vi "Write to Spreadsheet File.vi"(7 "1D data":dbl[](array[numeric]), 8 "error in (no error)":errorcluster, 9 "append to file? (F)":bool=TRUE, 11 "file path (dialog if empty)":path) -> (0 "error out":errorcluster)   [LabVIEW 2015]
uses:
  <vilib>/Utility/file.llb/Write Delimited Spreadsheet (DBL).vi
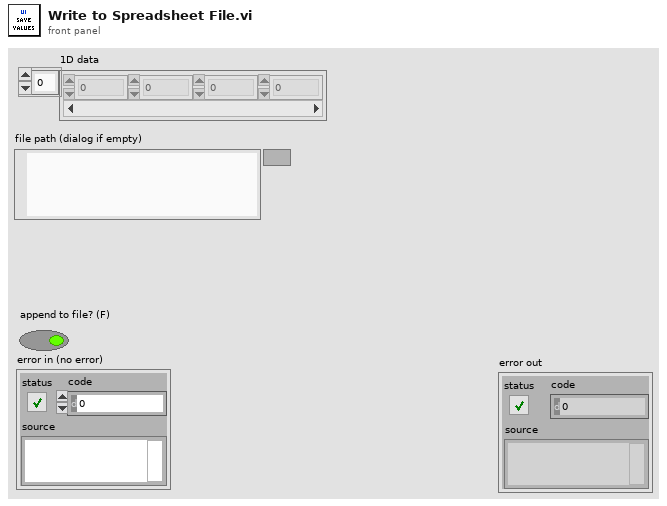
[diagram p1: front panel]
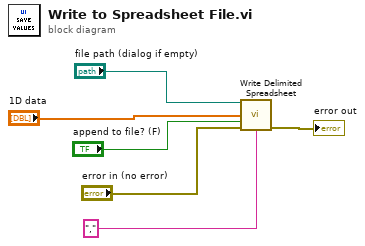
[diagram p0: block diagram]
diagram:
  n1 = call-poly <vilib>:"Write Delimited Spreadsheet.vi"("file path (dialog if empty)"="file path (dialog if empty)", "1D data"="1D data", "append to file? (F)"="append to file? (F)", "error in (no error)"="error in (no error)", "delimiter (\\t)"="," ("delimiter (\\t)")) -> ("error out"=→"error out":errorcluster)  [unwired: 9 in, 1 out]
